vi "DVR Qs limit test.vi"() -> ()   [LabVIEW 2021]
panel:
  in  "Numeric":i32=100000
  out "x-y":dbl format="%.8f"
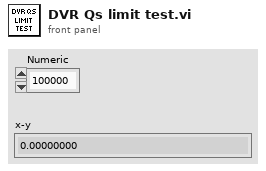
[diagram p1: front panel]
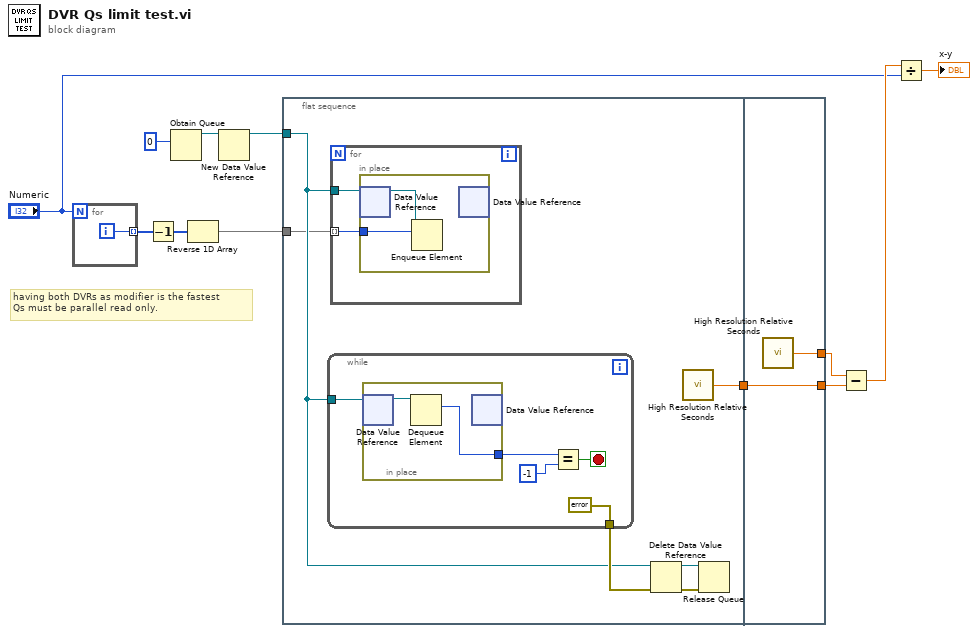
[diagram p0: block diagram]
diagram:
  # "having both DVRs as modifier is the fastest\nQs must be parallel read only."
  n1 = for {
    N: "Numeric" -> [_]
    tunnel: [w13] -> w10 mode=indexing
    i -> [w13]
  }
  n2 = Decrement(x=w10) -> (x-1=w11:i32[])
  n3 = Obtain Queue(element data type=0) -> (queue out=w4:refnum<queue>)  [unwired: 4 in, 2 out]
  n4 = Reverse 1D Array(array=w11) -> (reversed array=w1:i32[])
  n5 = New Data Value Reference(data value=w4) -> (data value reference=w2:refnum<data-value>)  [unwired: 1 in, 1 out]
  n6 = flat-sequence {
    tunnel: [w16] -> w8
    tunnel: w2 -> [w15]
    tunnel: w1 -> [w14]
    tunnel: [w32] -> w12
    tunnel: [w31] -> w9
    tunnel: w8 -> [w31]
    frame #0 {
      n7 = while {
        tunnel: w15 -> [w26]
        tunnel: [errorcluster {"status"=FALSE, "code"=0, "source"=""} ("error in (no error)")] -> w19
        stop <- w28 stop-if-true
        n8 = in-place {
          in-place-border: [w30] -> w24
          n9 = in-place-dvr #1(w26) -> (w29:refnum<queue>)  [unwired: 1 out]
          n10 = Dequeue Element(queue=w29) -> (element=w30:i32)  [unwired: 2 in, 3 out]
          n11 = in-place-dvr #1() -> ()  [unwired: 1 in, 2 out]
        }
        n12 = Equal?(x=w24, y=-1) -> (x = y?=w28:bool)
      }
      n13 = for {
        tunnel: w15 -> [w21]
        tunnel: w14 -> [w20] mode=indexing
        n14 = in-place {
          in-place-border: w20 -> [w22]
          n15 = in-place-dvr #2(w21) -> (w23:refnum<queue>)  [unwired: 1 out]
          n16 = Enqueue Element(queue=w23, element=w22) -> ()  [unwired: 2 in, 3 out]
          n17 = in-place-dvr #2() -> ()  [unwired: 1 in, 2 out]
        }
      }
      n18 = Delete Data Value Reference(data value reference=w15, error in=w19) -> (data value=w18:refnum<queue>, error out=w17:errorcluster)
      n19 = call <vilib>:"High Resolution Relative Seconds.vi"() -> ("relative seconds"=w16:dbl)
      n20 = Release Queue(queue=w18, error in (no error)=w17) -> ()  [unwired: 1 in, 3 out]
    }
    frame #1 {
      n21 = call <vilib>:"High Resolution Relative Seconds.vi"() -> ("relative seconds"=w32:dbl)
    }
  }
  n22 = Subtract(x=w12, y=w9) -> (x-y=w7:dbl)
  n23 = Divide(x=w7, y="Numeric") -> (x/y=→"x-y":dbl)
